vi "SERIAL_StreamProcessor.vi"() -> ()   [LabVIEW 2014, in "navX-MXP IMU.lvlib"]
uses:
  navX-MXP IMU.lvlib
  COMMON/TypeDefs/navX Device TypeDef.ctl
  COMMON/TypeDefs/Value TypeDefs/navX Interface Protocol.ctl
  <vilib>/Rock Robotics/WPI/SPI/WPI_SPIDevRef.ctl
  <vilib>/Rock Robotics/SystemInterfaces/Typedef/FPGA_TypedefDigitalModule.ctl
  <vilib>/Rock Robotics/SystemInterfaces/spilib/spi_bus.ctl
  <vilib>/Rock Robotics/WPI/I2C/WPI_I2CDevRef.ctl
  <vilib>/Rock Robotics/SystemInterfaces/i2clib/i2c_bus.ctl
  <vilib>/Rock Robotics/WPI/SerialPort/WPI_SerialPortRef.ctl
  COMMON/TypeDefs/Data TypeDefs/navX Board Information.ctl
  COMMON/TypeDefs/Value TypeDefs/navX NAVX_BOARD_CAPABILITY.ctl
  COMMON/TypeDefs/Value TypeDefs/navX NAVX_BOARD_YAW_AXIS.ctl
  COMMON/TypeDefs/Data TypeDefs/navX Status Data.ctl
  COMMON/TypeDefs/Value TypeDefs/navX NAVX_OP_STATUS.ctl
  COMMON/TypeDefs/Value TypeDefs/navX NAVX_CAL_STATUS.ctl
  COMMON/TypeDefs/Value TypeDefs/navX NAVX_SENSOR_STATUS.ctl
  COMMON/TypeDefs/Data TypeDefs/navX Offsets Data.ctl
  COMMON/TypeDefs/Value TypeDefs/navX Update Rate.ctl
  COMMON/TypeDefs/Value TypeDefs/navX Serial Mode.ctl
  <vilib>/Platform/TimedLoop/XDataNode/timing_clust.ctl
  <vilib>/Platform/TimedLoop/XDataNode/nitl_modes.ctl
  <vilib>/Platform/TimedLoop/XDataNode/wakeup.ctl
  COMMON/TypeDefs/Value TypeDefs/navX Device Registers.ctl
  <vilib>/Rock Robotics/SystemInterfaces/Utilities/FPGA_UtilitiesRead LocalTime.vi
  <vilib>/platform/TimedLoop/XDataNode/XDataNode.xnode
  <vilib>/Platform/TimedLoop/XDataNode/XDNodeRunTimeDep.lvlib
panel:
  in  "navX Device TypeDef":T1={"navX Interface Protocol"=enum."SPI", "navX Interface Protocol TypeDefs"={"SPIDevRef"={"DevStatus"={"status"=FALSE, "code"=0, "source"=""}, "Handle"=0, "Controller"=enum."Controller 1", "SPI Bus"=enum."SPI On-Board, CS0"}, "I2CDevRef"={"DevStatus"={"status"=FALSE, "code"=0, "source"=""}, "Controller"=enum."Controller 1", "Device Address"=0, "Handle"=0, "I2C Bus"=enum."Invalid"}, "SerialPortRef"={"DevStatus"={"status"=FALSE, "code"=0, "source"=""}, "Serial Port Name"=""}}, "navX System Information"={"Board Information"={"WhoAmI (50 | 0x32)"=0, "Board Revision"=0, "Firmware Major Version"=0, "Firmware Minor Version"=0, "NAVX_BOARD_CAPABILITY"={"OMNIMOUNT"=FALSE, "YAW_RESET"=FALSE, "VEL_AND_DISP"=FALSE}, "NAVX_BOARD_YAW_AXIS"={"BOARD_YAW_AXIS_UP"=FALSE, "BOARD_YAW_AXIS"=0}}, "Status"={"Update Rate Hz"=0, "Accelerometer Full-Scale Range"=0, "Gyro Full-Scale Range"=0, "NAVX_OP_STATUS"=0, "NAVX_CAL_STATUS"=0, "NAVX_SELFTEST_STATUS"=0, "NAVX_SENSOR_STATUS"={"MOVING"=FALSE, "YAW_STABLE"=FALSE, "MAG_DISTURBANCE"=FALSE, "ALTITUDE_VALID"=FALSE, "SEALEVEL_PRESS_SET"=FALSE, "FUSED_HEADING_VALID"=FALSE}}, "Offsets"={"Yaw"=0.0, "Quat W"=0.0, "Quat X"=0.0, "Quat Y"=0.0, "Quat Z"=0.0}, "LastSampleTimestamp"=0.0, "LastSampleValid"=FALSE}, "navX Common Information"={"Update Rate (4Hz-60Hz)"=50, "refnum name"="", "error"={"status"=FALSE, "code"=0, "source"=""}, "LastFPGATimestamp"=0.0, "Reboot Detected"=FALSE}, "Serial Protocol Extra"={"Loop VI Refnum"=refnum, "Nav6Mode (YPR)"=enum."Raw"}} {"navX Common Information"."Update Rate (4Hz-60Hz)" min=4 max=60 step=1; "navX System Information"."Status"."NAVX_OP_STATUS" items=["INITIALIZING", "SELFTEST_IN_PROGRESS", "ERROR", "IMU_AUTOCAL_IN_PROGRESS", "NORMAL"]; "navX System Information"."Status"."NAVX_CAL_STATUS" items=["IMU_CAL_STATE_MASK"=3, "IMU_CAL_INPROGRESS"=0, "IMU_CAL_ACCUMULATE"=1, "IMU_CAL_COMPLETE"=2, "MAG_CAL_COMPLETE"=4, "BARO_CAL_COMPLETE"=8]; "navX Interface Protocol TypeDefs"."I2CDevRef"."Device Address" format="%.0x"}
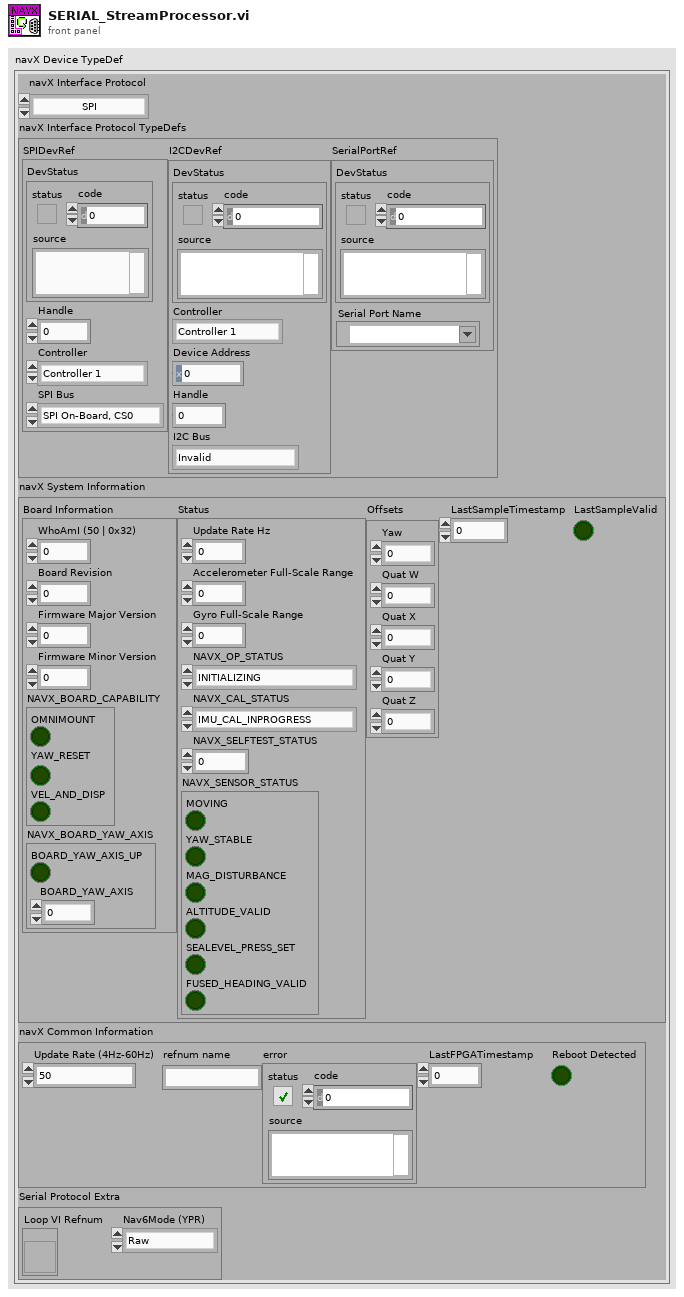
[diagram p1: front panel]
types:
  T1 = typedef "navX-MXP IMU.lvlib/navX Device TypeDef.ctl" = cluster{"navX Interface Protocol":T2, "navX Interface Protocol TypeDefs":cluster{"SPIDevRef":T3, "I2CDevRef":T6, "SerialPortRef":T8}, "navX System Information":cluster{"Board Information":T9, "Status":T12, "Offsets":T16, "LastSampleTimestamp":dbl, "LastSampleValid":bool}, "navX Common Information":cluster{"Update Rate (4Hz-60Hz)":T17, "refnum name":string, "error":errorcluster, "LastFPGATimestamp":dbl, "Reboot Detected":bool}, "Serial Protocol Extra":cluster{"Loop VI Refnum":refnum<vi>, "Nav6Mode (YPR)":T18}}
  T2 = typedef "navX-MXP IMU.lvlib/navX Interface Protocol.ctl" = enum16{"SPI", "I2C", "SERIAL"}
  T3 = typedef "WPI_SPIDevRef.ctl" = cluster{"DevStatus":errorcluster, "Handle":i32, "Controller":T4, "SPI Bus":T5}
  T4 = typedef "FPGA_TypedefDigitalModule.ctl" = enum16{"Controller 1"}
  T5 = typedef "spi_bus.ctl" = enum16{"SPI On-Board, CS0", "SPI On-Board, CS1", "SPI On-Board, CS2", "SPI On-Board, CS3", "SPI MXP", "Invalid"}
  T6 = typedef "WPI_I2CDevRef.ctl" = cluster{"DevStatus":errorcluster, "Controller":T4, "Device Address":u8, "Handle":i32, "I2C Bus":T7}
  T7 = typedef "i2c_bus.ctl" = enum16{"I2C On-Board", "I2C MXP", "Invalid"}
  T8 = typedef "WPI_SerialPortRef.ctl" = cluster{"DevStatus":errorcluster, "Serial Port Name":refnum<visa-resource-name>}
  T9 = typedef "navX-MXP IMU.lvlib/navX Board Information.ctl" = cluster{"WhoAmI (50 | 0x32)":u8, "Board Revision":u8, "Firmware Major Version":u8, "Firmware Minor Version":u8, "NAVX_BOARD_CAPABILITY":T10, "NAVX_BOARD_YAW_AXIS":T11}
  T10 = typedef "navX-MXP IMU.lvlib/navX NAVX_BOARD_CAPABILITY.ctl" = cluster{"OMNIMOUNT":bool, "YAW_RESET":bool, "VEL_AND_DISP":bool}
  T11 = typedef "navX-MXP IMU.lvlib/navX NAVX_BOARD_YAW_AXIS.ctl" = cluster{"BOARD_YAW_AXIS_UP":bool, "BOARD_YAW_AXIS":u8}
  T12 = typedef "navX-MXP IMU.lvlib/navX Status Data.ctl" = cluster{"Update Rate Hz":u8, "Accelerometer Full-Scale Range":u8, "Gyro Full-Scale Range":u16, "NAVX_OP_STATUS":T13, "NAVX_CAL_STATUS":T14, "NAVX_SELFTEST_STATUS":u8, "NAVX_SENSOR_STATUS":T15}
  T13 = typedef "navX-MXP IMU.lvlib/navX NAVX_OP_STATUS.ctl" = u8
  T14 = typedef "navX-MXP IMU.lvlib/navX NAVX_CAL_STATUS.ctl" = u8
  T15 = typedef "navX-MXP IMU.lvlib/navX NAVX_SENSOR_STATUS.ctl" = cluster{"MOVING":bool, "YAW_STABLE":bool, "MAG_DISTURBANCE":bool, "ALTITUDE_VALID":bool, "SEALEVEL_PRESS_SET":bool, "FUSED_HEADING_VALID":bool}
  T16 = typedef "navX-MXP IMU.lvlib/navX Offsets Data.ctl" = cluster{"Yaw":dbl, "Quat W":dbl, "Quat X":dbl, "Quat Y":dbl, "Quat Z":dbl}
  T17 = typedef "navX-MXP IMU.lvlib/navX Update Rate.ctl" = u8
  T18 = typedef "navX-MXP IMU.lvlib/navX Serial Mode.ctl" = enum16{"Raw", "Processed"}
  T19 = typedef "XDNodeRunTimeDep.lvlib/timing_clust.ctl" = cluster{"Expected End [f-1]":u64, "Actual End [f-1]":u64, "Finished Late? [f-1]":bool, "Expected End [i-1]":u64, "Actual End [i-1]":u64, "Finished Late? [i-1]":bool, "Expected Start [i]":u64, "Actual Start [i]":u64, "Expected Start [f]":u64, "Actual Start [f]":u64, "Source Name":string, "Structure Name":string, "Period":i64, "Deadline":i64, "Offset":i64, "Start":i64, "Priority":i32, "Timeout":i32, "Mode":T20, "Wakeup Reason":T21, "Error":errorcluster, "Source Type":string, "Secondary Source Type":string, "Global End Time":u64, "Global Start Time":u64, "Frame Duration":u64, "Iteration Duration":u64, "Assigned CPU":i32, "I/O Scan Engine Mode":u32}
  T20 = typedef "XDNodeRunTimeDep.lvlib/nitl_modes.ctl" = enum32{"No Change", "Process missed periods, maintain original phase", "Discard missed periods, maintain original phase", "Process missed periods, ignore original phase", "Discard missed periods, ignore original phase"}
  T21 = typedef "XDNodeRunTimeDep.lvlib/wakeup.ctl" = enum32{"Normal", "Aborted", "Asynchronous wakeup", "Timing source error", "Timed loop error", "Timeout"}
  T22 = typedef "navX-MXP IMU.lvlib/navX Device Registers.ctl" = u8
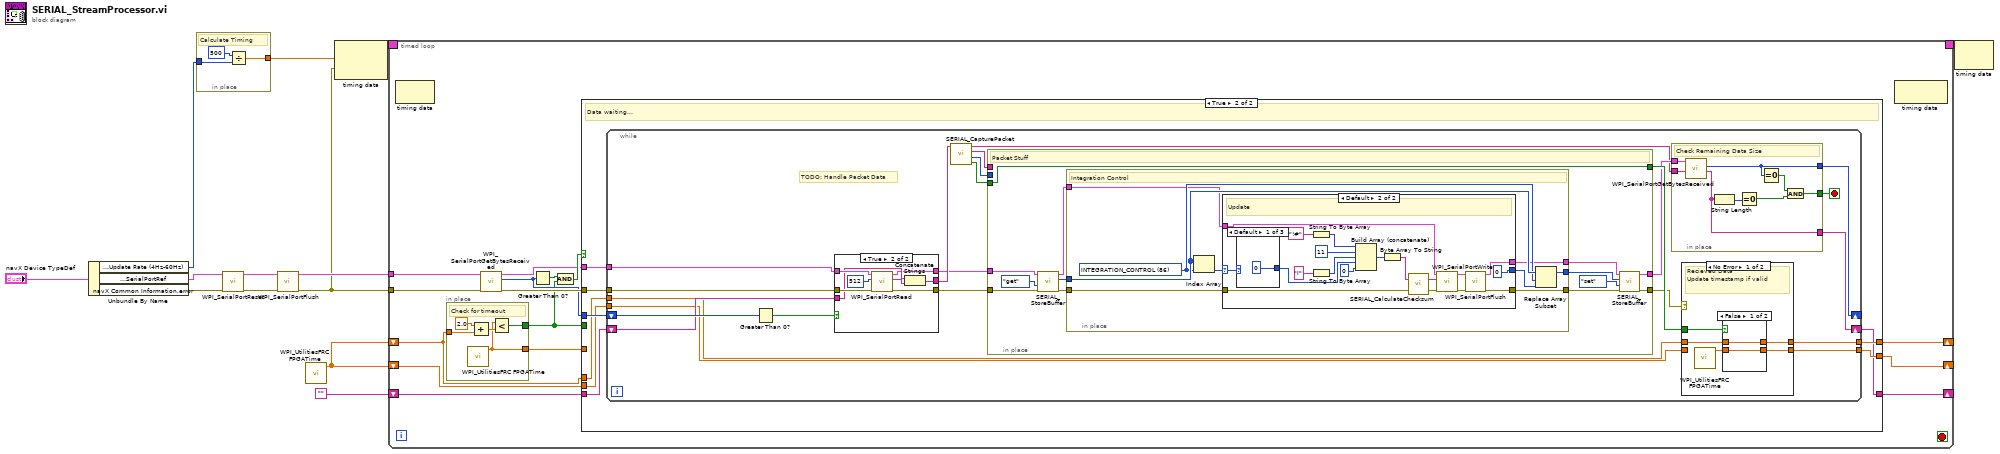
[diagram p0: block diagram]
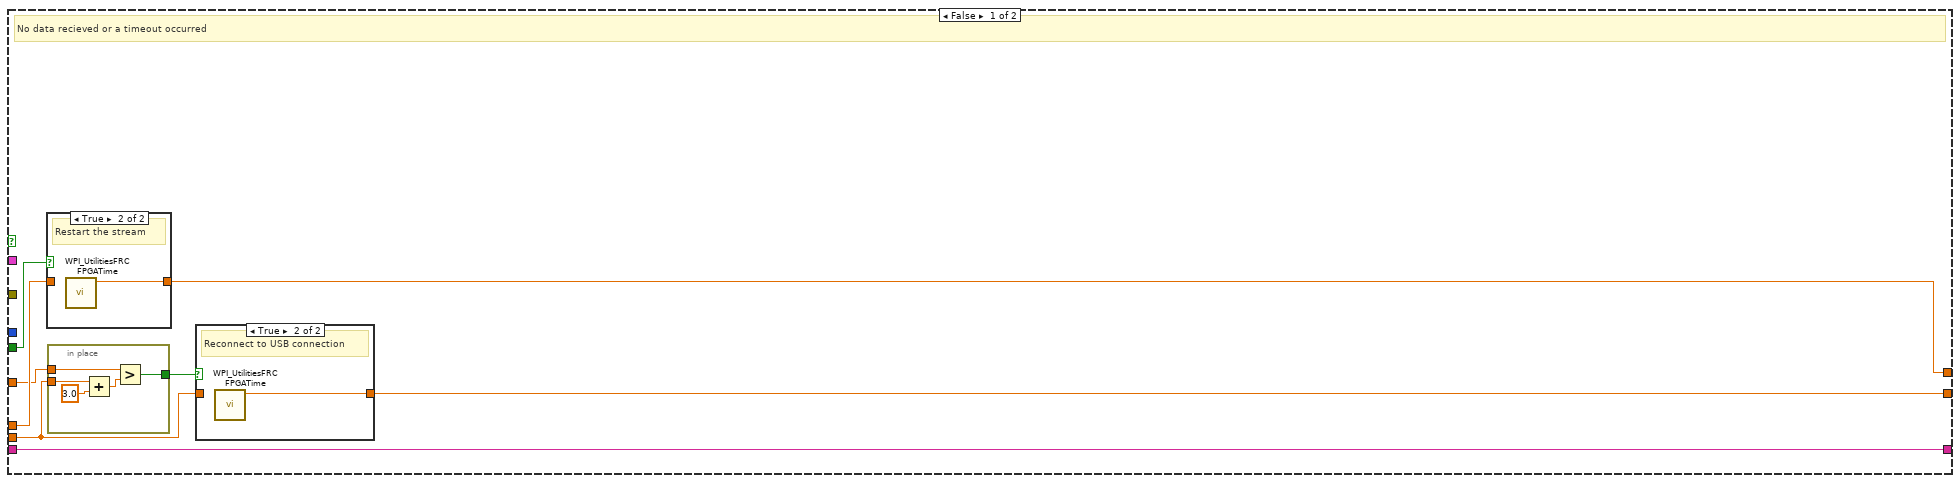
[diagram p2: hidden frame]
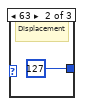
[diagram p8: hidden frame]
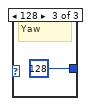
[diagram p9: hidden frame]
diagram:
  n1 = Unbundle By Name("navX Device TypeDef") -> ("navX Common Information.Update Rate (4Hz-60Hz)"=w1:T17, "navX Interface Protocol TypeDefs.SerialPortRef"=w4:T8, "navX Common Information.error"=w3:errorcluster)
  n2 = in-place {
    in-place-border: w1 -> [w15]
    in-place-border: [w14] -> w2
    # "Calculate Timing"
    n3 = Divide(x=500, y=w15) -> (x/y=w14:dbl)
  }
  n4 = call <vilib>:"WPI_SerialPortReset.vi"("error in (no error)"=w3, "SerialPortRef"=w4) -> ("error out"=w11:errorcluster, "SerialPortRef"=w10:T8)  [unwired: 8 in]
  n5 = call <vilib>:"WPI_SerialPortFlush.vi"("error in (no error)"=w11, "SerialPortRef"=w10) -> ("error out"=w8:errorcluster, "SerialPortRef"=w9:T8)  [unwired: 8 in]
  n6 = call <vilib>:"WPI_UtilitiesFRC FPGATime.vi"() -> ("FPGA Time"=w7:dbl)  [unwired: 10 in, 1 out]
  n7 = node-c288(w2, w8) -> (w13:T19)
  n8 = timed-loop {
    timing: w13 -> [_]
    timing-out: [_] -> w12
    tunnel: w9 -> [w26]
    tunnel: w8 -> [w31]
    shift-right: [w22] -> _
    shift-left: w7 -> [w23]
    shift-right: [w21] -> _
    shift-left: w7 -> [w20]
    shift-right: [w17] -> _
    shift-left: "" -> [w24]
    stop <- _ stop-if-true
    n9 = node-c288() -> ()  [unwired: 1 in, 1 out]
    n10 = in-place {
      in-place-border: w23 -> [w158]
      in-place-border: [w156] -> w19
      in-place-border: [w155] -> w18
      # "Check for timeout"
      n11 = call <vilib>:"WPI_UtilitiesFRC FPGATime.vi"() -> ("FPGA Time"=w155:dbl)  [unwired: 10 in, 1 out]
      n12 = Add(x=2.0, y=w158) -> (x+y=w157:dbl)
      n13 = Less?(x=w155, y=w157) -> (x < y?=w156:bool)
    }
    n14 = call <vilib>:"WPI_SerialPortGetBytesReceived.vi"("error in (no error)"=w31, "SerialPortRef"=w26) -> ("error out"=w27:errorcluster, "Bytes at Port"=w25:u32, "SerialPortRef"=w28:T8)  [unwired: 7 in]
    n15 = Greater Than 0?(x=w25) -> (x > 0?=w30:bool)
    n16 = Compound Arithmetic op=AND(w30, w19) -> (w29:bool)
    n17 = case shown="True" w29 {
      tunnel: w28 -> [_ w56]
      tunnel: w27 -> [_ w55]
      tunnel: w25 -> [_ w57]
      tunnel: w24 -> [w32 w54]
      tunnel: w23 -> [w38 w53]
      tunnel: [w33 w52] -> w22
      tunnel: [w34 w51] -> w21
      tunnel: w20 -> [w35 w50]
      tunnel: w19 -> [w39 _]
      tunnel: w18 -> [w37 _]
      tunnel: [w32 w49] -> w17
      frame False {
        # "No data recieved or a timeout occurred"
        n18 = case shown="True" w39 {
          tunnel: [w47 w48] -> w33
          tunnel: w38 -> [w47 _]
          frame False {
          }
          frame True {
            # "Restart the stream"
            n19 = call <vilib>:"WPI_UtilitiesFRC FPGATime.vi"() -> ("FPGA Time"=w48:dbl)  [unwired: 10 in, 1 out]
          }
        }
        n20 = in-place {
          in-place-border: w37 -> [w42]
          in-place-border: [w41] -> w36
          in-place-border: w35 -> [w40]
          n21 = Add(x=w40, y=3.0) -> (x+y=w43:dbl)
          n22 = Greater?(x=w42, y=w43) -> (0:w41:bool)
        }
        n23 = case shown="True" w36 {
          tunnel: [w45 w46] -> w34
          tunnel: w35 -> [w45 _]
          frame False {
          }
          frame True {
            # "Reconnect to USB connection"
            n24 = call <vilib>:"WPI_UtilitiesFRC FPGATime.vi"() -> ("FPGA Time"=w46:dbl)  [unwired: 10 in, 1 out]
          }
        }
      }
      frame True {
        # "Data waiting..."
        n25 = while {
          shift-right: [w61] -> _
          shift-left: w57 -> [w79]
          tunnel: w56 -> [w77]
          tunnel: w55 -> [w76]
          shift-right: [w58] -> w49
          shift-left: w54 -> [w75]
          tunnel: w53 -> [w67]
          tunnel: [w66] -> w52
          tunnel: [w65] -> w51
          tunnel: w50 -> [w64]
          stop <- w60 stop-if-true
          # "TODO: Handle Packet Data"
          n26 = Greater Than 0?(x=w79) -> (x > 0?=w78:bool)
          n27 = case shown="True" w78 {
            tunnel: w77 -> [w144 w153]
            tunnel: w76 -> [w145 w152]
            tunnel: w75 -> [w146 w150]
            tunnel: [w146 w149] -> w74
            tunnel: [w145 w148] -> w69
            tunnel: [w144 w147] -> w70
            frame False {
            }
            frame True {
              n28 = call <vilib>:"WPI_SerialPortRead.vi"("error in (no error)"=w152, "Num Bytes to Read"=u32 512, "SerialPortRef"=w153) -> ("error out"=w148:errorcluster, "Buffer"=w151:string, "SerialPortRef"=w147:T8)  [unwired: 6 in]
              n29 = Concatenate Strings(w150, w151) -> (w149:string)
            }
          }
          n30 = call "SERIAL_CapturePacket.vi"("Stream"=w74) -> ("Packet Located"=w71:bool, "Packet Length"=w72:i32, "Packet"=w73:string, "Stream"=w59:string)  [unwired: 7 in]
          n31 = in-place {
            in-place-border: w73 -> [_]
            in-place-border: w72 -> [_]
            in-place-border: w71 -> [w97]
            in-place-border: w70 -> [w109]
            in-place-border: w69 -> [w106]
            in-place-border: [w105] -> w63
            in-place-border: [w98] -> w62
            in-place-border: [w97] -> w68
            # "Packet Stuff"
            n32 = call "SERIAL_StoreBuffer.vi"("error in (no error)"=w106, "Access Type"=enum16{"set", "get", "delete"}."get", "SerialPortRef"=w109) -> ("error out"=w103:errorcluster, "navX Data"=w104:u8[], "SerialPortRef"=w100:T8)  [unwired: 6 in]
            n33 = in-place {
              in-place-border: w104 -> [w117]
              in-place-border: [w114] -> w101
              in-place-border: [w113] -> w99
              in-place-border: w100 -> [w112]
              in-place-border: w103 -> [w111]
              in-place-border: [w110] -> w102
              w116 = T22 86 items=["WHOAMI"=0, "HW_REV"=1, "FW_VER_MAJOR"=2, "FW_VER_MINOR"=3, "UPDATE_RATE_HZ"=4, "ACCEL_FSR_G"=5, "GYRO_FSR_DPS"=6, "OP_STATUS"=8, "CAL_STATUS"=9, "SELFTEST_STATUS"=10, "CAPABILITY_FLAGS_L"=11, "CAPABILITY_FLAGS_H"=12, "SENSOR_STATUS"=16, "TIMESTAMP"=18, "YAW"=22, "PITCH"=24, "ROLL"=26, "HEADING"=28, "FUSED_HEADING"=30, "ALTITUDE_I"=32, "ALTITUDE_D"=34, "LINERA_ACC_X"=36, "LINERA_ACC_Y"=38, "LINERA_ACC_Z"=40, "QUAT_W"=42, "QUAT_X"=44, "QUAT_Y"=46, "QUAT_Z"=48, "MPU_TEMP_C"=50, "GYRO_X"=52, "GYRO_Y"=54, "GYRO_Z"=56, "ACC_X"=58, "ACC_Y"=60, "ACC_Z"=62, "MAG_X"=64, "MAG_Y"=66, "MAG_Z"=68, "PRESSURE_I"=70, "PRESSURE_D"=72, "PRESSURE_TEMP"=74, "YAW_OFFSET"=76, "QUAT_OFFSET_W"=78, "QUAT_OFFSET_X"=80, "QUAT_OFFSET_Y"=82, "QUAT_OFFSET_Z"=84, "INTEGRATION_CONTROL"=86, "VELOCITY_X"=88, "VELOCITY_Y"=92, "VELOCITY_Z"=96, "DISPLACMENT_X"=100, "DISPLACMENT_Y"=104, "DISPLACEMENT_Z"=108] ("Device Register")
              # "Integration Control"
              n34 = Index Array(array=w117, index=w116) -> (element=w118:u8)
              n35 = case shown="Default" w118 {
                selector: w118 -> [w121 w139]
                tunnel: [w121 0] -> w115
                tunnel: [w120 w125] -> w113
                tunnel: [w119 w124] -> w110
                tunnel: w112 -> [w120 w123]
                tunnel: w111 -> [w119 w122]
                frame 0 {
                }
                frame Default {
                  # "Update"
                  n36 = case shown="Default" w139 {
                    tunnel: [0 127 128] -> w132
                    frame Default {
                    }
                    frame 63 {
                      # "Displacement"
                    }
                    frame 128 {
                      # "Yaw"
                    }
                  }
                  n37 = String To Byte Array(string="!#") -> (unsigned byte array=w136:u8[])
                  n38 = String To Byte Array(string="I" ("format string")) -> (unsigned byte array=w134:u8[])
                  n39 = Build Array (concatenate)(w136, 11, w134, w132, 0) -> (w131:i32[])
                  n40 = Byte Array To String(unsigned byte array=w131) -> (string=w130:string)
                  n41 = call "SERIAL_CalculateChecksum.vi"("error in"=w122, "Content"=w130) -> ("error out"=w126:errorcluster, "Teminated Content"=w127:string)
                  n42 = call <vilib>:"WPI_SerialPortWrite.vi"("error in (no error)"=w126, "Buffer"=w127, "SerialPortRef"=w123) -> ("error out"=w129:errorcluster, "SerialPortRef"=w128:T8)  [unwired: 6 in, 1 out]
                  n43 = call <vilib>:"WPI_SerialPortFlush.vi"("error in (no error)"=w129, "SerialPortRef"=w128) -> ("error out"=w124:errorcluster, "SerialPortRef"=w125:T8)  [unwired: 8 in]
                }
              }
              n44 = Replace Array Subset(array=w117, new element=w115, index=w116) -> (w114:u8[])
            }
            n45 = call "SERIAL_StoreBuffer.vi"("error in (no error)"=w102, "Access Type"=enum16{"set", "get", "delete"}."set", "navX Data"=w101, "SerialPortRef"=w99) -> ("error out"=w105:errorcluster, "SerialPortRef"=w98:T8)  [unwired: 5 in, 1 out]
          }
          n46 = in-place {
            in-place-border: w62 -> [w86]
            in-place-border: [w85] -> w61
            in-place-border: [w80] -> w58
            in-place-border: [w82] -> w60
            in-place-border: w59 -> [w80]
            # "Check Remaining Data Size"
            n47 = call <vilib>:"WPI_SerialPortGetBytesReceived.vi"("SerialPortRef"=w86) -> ("Bytes at Port"=w85:u32)  [unwired: 8 in, 2 out]
            n48 = String Length(string=w80) -> (length=w84:i32)
            n49 = Equal To 0?(x=w84) -> (x = 0?=w81:bool)
            n50 = Equal To 0?(x=w85) -> (x = 0?=w83:bool)
            n51 = Compound Arithmetic op=AND(w83, w81) -> (w82:bool)
          }
          n52 = case shown="No Error" w63 {
            tunnel: [w91 w96] -> w66
            tunnel: w67 -> [w90 w96]
            tunnel: w64 -> [_ w95]
            tunnel: [w89 w95] -> w65
            tunnel: w68 -> [w87 _]
            frame No Error {
              # "Recieved Data\nUpdate timestamp if valid"
              n53 = call <vilib>:"WPI_UtilitiesFRC FPGATime.vi"() -> ("FPGA Time"=w88:dbl)  [unwired: 10 in, 1 out]
              n54 = case shown="False" w87 {
                tunnel: [w93 w94] -> w91
                tunnel: w90 -> [w93 _]
                tunnel: [w92 w94] -> w89
                tunnel: w88 -> [w92 w94]
                frame False {
                }
                frame True {
                }
              }
            }
            frame Error {
            }
          }
        }
      }
    }
    n55 = node-c288() -> ()  [unwired: 1 in, 1 out]
  }
  n56 = node-c288(w12) -> ()  [unwired: 1 out]
